vi "parse_asyncChFixedSize.vi"(8 "error in (no error)":errorcluster, 9 "ChannelInfo":T2, 10 "AcquisitionStart":T4, 11 "Package String":string) -> (0 "error out":errorcluster, 1 "Timebase\nFrequency":dbl, 3 "Data":T1)   [LabVIEW 2020, in "OXYGEN_Datastream.lvlib"]
uses:
  OXYGEN_Datastream.lvlib
  TypeDefs/AcqInfo_AcquisitionStart.ctl
  TypeDefs/AcqInfo_AcquisitionStart_nanoseconds.ctl
  TypeDefs/ChannelInfo.ctl
  TypeDefs/ChannelInfo_Scaling.ctl
  TypeDefs/DataPoint_Variant.ctl
  parse_dataString.vi
panel:
  out "Pckg Info":u32
  out "remaining data":string
  out "Data samples raw":string
  out "#Samples":u32
  out "Dimension":u32
  out "Sample data type":u32
  out "Package size":u32
  # "3 --> sync channel with fixed sample rate"
  # "4 --> sint24"
  # "1 -- Scalar"
  # "= (pckg size - 32) / 3"
  # "--> must be empty!"
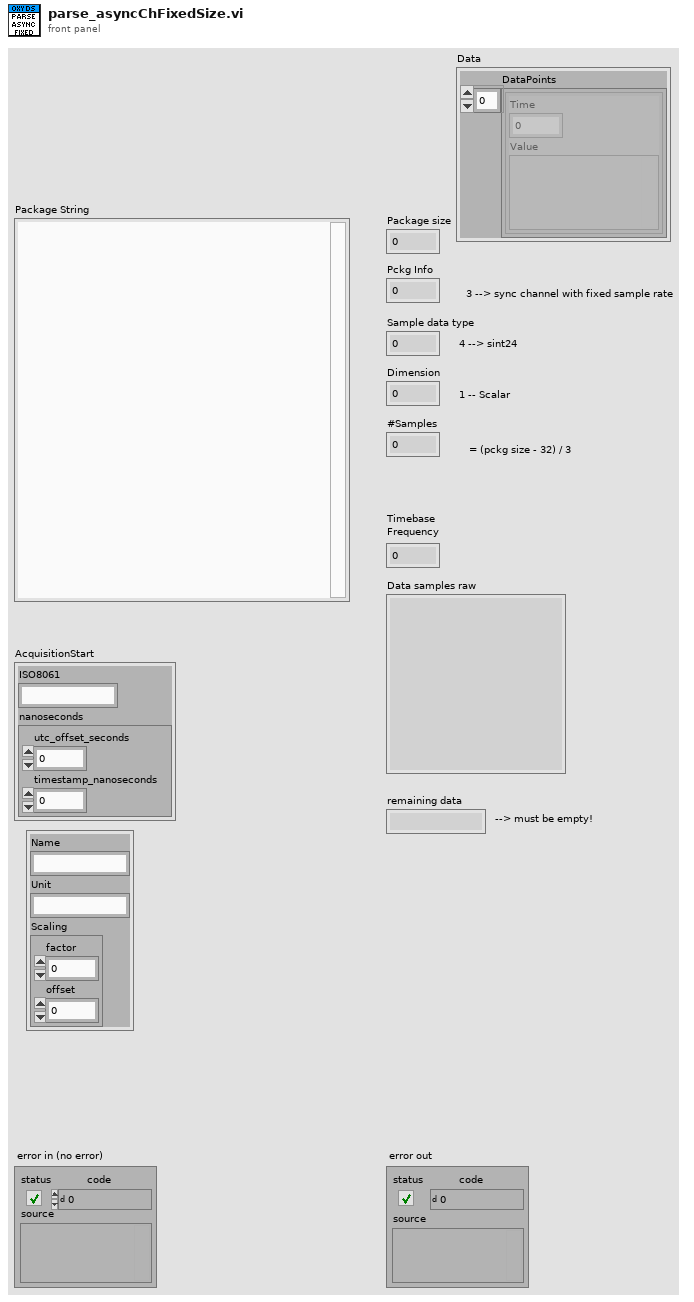
[diagram p1: front panel]
types:
  T1 = typedef "OXYGEN_Datastream.lvlib/DataPoint_Variant.ctl" = cluster{"DataPoints":cluster{"Time":dbl, "Value":variant}[]}
  T2 = typedef "OXYGEN_Datastream.lvlib/ChannelInfo.ctl" = cluster{"Name":string, "Unit":string, "Scaling":T3}
  T3 = typedef "OXYGEN_Datastream.lvlib/ChannelInfo_Scaling.ctl" = cluster{"factor":dbl, "offset":dbl}
  T4 = typedef "OXYGEN_Datastream.lvlib/AcqInfo_AcquisitionStart.ctl" = cluster{"ISO8061":string, "nanoseconds":T5}
  T5 = typedef "OXYGEN_Datastream.lvlib/AcqInfo_AcquisitionStart_nanoseconds.ctl" = cluster{"utc_offset_seconds":i64, "timestamp_nanoseconds":i64}
  T6 = enum16{"big-endian, network order", "native, host order", "little-endian"}
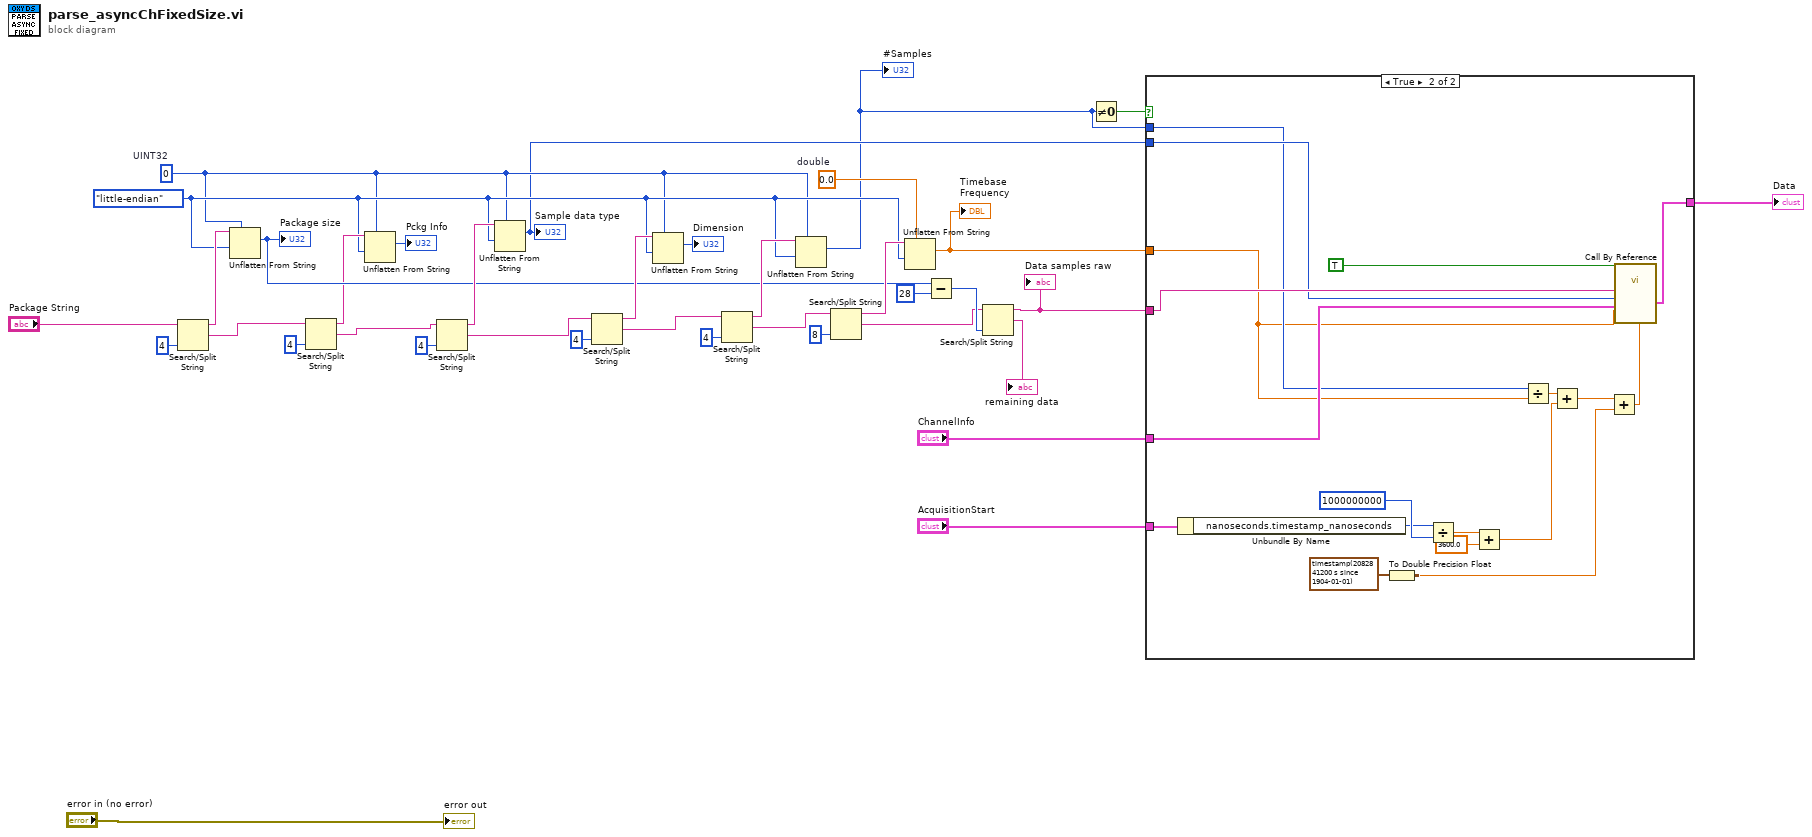
[diagram p0: block diagram]
diagram:
  w7 = 0.0  # double
  w12 = u32 0  # UINT32
  w13 = T6."little-endian" ("byte order (0:big-endian, network order)")
  n1 = Search/Split String(string="Package String", offset (0)=4) -> (substring before match=w31:string, match + rest of string=w16:string)  [unwired: 1 in, 1 out]
  n2 = Unflatten From String(type=w12, binary string=w31, byte order (0:big-endian, network order)=w13) -> (value=w22:u32)  [unwired: 2 in, 2 out]
  "Package size" <- w22
  n3 = Search/Split String(string=w16, offset (0)=4) -> (substring before match=w15:string, match + rest of string=w14:string)  [unwired: 1 in, 1 out]
  n4 = Unflatten From String(type=w12, binary string=w15, byte order (0:big-endian, network order)=w13) -> (value=→"Pckg Info":u32)  [unwired: 2 in, 2 out]
  n5 = Search/Split String(string=w14, offset (0)=4) -> (substring before match=w29:string, match + rest of string=w32:string)  [unwired: 1 in, 1 out]
  n6 = Unflatten From String(type=w12, binary string=w29, byte order (0:big-endian, network order)=w13) -> (value=w9:u32)  [unwired: 2 in, 2 out]
  "Sample data type" <- w9
  n7 = Search/Split String(string=w32, offset (0)=4) -> (substring before match=w27:string, match + rest of string=w30:string)  [unwired: 1 in, 1 out]
  n8 = Unflatten From String(type=w12, binary string=w27, byte order (0:big-endian, network order)=w13) -> (value=→"Dimension":u32)  [unwired: 2 in, 2 out]
  n9 = Search/Split String(string=w30, offset (0)=4) -> (substring before match=w26:string, match + rest of string=w24:string)  [unwired: 1 in, 1 out]
  n10 = Unflatten From String(type=w12, binary string=w26, byte order (0:big-endian, network order)=w13) -> (value=w1:u32)  [unwired: 2 in, 2 out]
  "#Samples" <- w1
  n11 = Search/Split String(string=w24, offset (0)=8) -> (substring before match=w23:string, match + rest of string=w6:string)  [unwired: 1 in, 1 out]
  n12 = Unflatten From String(type=w7, binary string=w23, byte order (0:big-endian, network order)=w13) -> (value=w4:dbl)  [unwired: 2 in, 2 out]
  "Timebase\nFrequency" <- w4
  n13 = Subtract(x=w22, y=u32 28) -> (x-y=w20:u32)
  n14 = Search/Split String(string=w6, offset (0)=w20) -> (substring before match=w10:string, match + rest of string=→"remaining data":string)  [unwired: 1 in, 1 out]
  "Data samples raw" <- w10
  n15 = Not Equal To 0?(x=w1) -> (x != 0?=w3:bool)
  n16 = case shown="True" w3 {
    tunnel: w10 -> [_ w55]
    tunnel: w9 -> [_ w54]
    tunnel: "AcquisitionStart" -> [_ w52]
    tunnel: "ChannelInfo" -> [_ w50]
    tunnel: w4 -> [_ w39]
    tunnel: [_ w42] -> w2
    tunnel: w1 -> [_ w40]
    frame False {
    }
    frame True {
      n17 = Unbundle By Name(w52) -> ("nanoseconds.timestamp_nanoseconds"=w47:i64)
      n18 = To Double Precision Float(number=timestamp(2082841200 s since 1904-01-01)) -> (double precision float=w46:dbl)
      n19 = Divide(x=w47, y=i64 1000000000) -> (x/y=w49:dbl)
      n20 = Add(x=w49, y=3600.0) -> (x+y=w45:dbl)
      n21 = Divide(x=w40, y=w39) -> (x/y=w43:dbl)
      n22 = Add(x=w43, y=w45) -> (x+y=w44:dbl)
      n23 = Add(x=w44, y=w46) -> (x+y=w41:dbl)
      n24 = call-by-ref "?"("Timestamp"=w41, "Timebase Frequency"=w39, "Includes Timestamp?"=TRUE, "ChannelInfo"=w50, "Data Type"=w54, "Data String"=w55) -> ("Data"=w42:T1)  [unwired: 6 in, 3 out]
    }
  }
  "Data" <- w2
  "error out" <- "error in (no error)"
